vi "Teleop.vi"(10 "Match Info":T1={"Autonomous Elapsed Seconds"=0.0, "TeleOp Elapsed Seconds"=0.0, "Disabled Elapsed Seconds"=0.0, "Visited Autonomous"=FALSE, "Visited TeleOp"=FALSE, "Visited Disabled"=FALSE, "Autonomous Settings"={"Autonomous Style"=enum."Independent", "VI Refnum"=refnum}}, 11 "Call Context":T2=enum."Execute") -> ()   [LabVIEW 2013]
doc: "This VI is called for each TeleOp packet received from the DS where the robot is not disabled. It is often used to read from the joysticks and update I/O or to update setpoints for timed control loops. It should complete and return within 20 milliseconds or it may miss DS packets."
uses:
  <vilib>/Rock Robotics/WPI/DriverStation/WPI_DriverStationDerivedRobotMode.ctl
  <vilib>/Rock Robotics/WPI/DriverStation/WPI_DriverStationMatch Info.ctl
  Robot Global Data.vi
  <vilib>/Rock Robotics/WPI/Joystick/WPI_JoystickGetSetRefNum.vi
  <vilib>/Rock Robotics/WPI/RobotDrive/WPI_RobotDriveGetSetRefNum.vi
panel:
  in  "Joystick Mult Slow":dbl=0.5
  in  "Joystick Mult":dbl=1.0
  in  "Rest Speed r/s":dbl=15.0 min=0.0 max=0.7 step=0.05
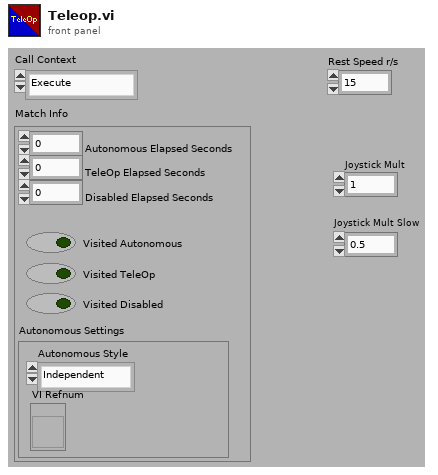
[diagram p1: front panel]
types:
  T1 = typedef "WPI_DriverStationMatch Info.ctl" = cluster{"Autonomous Elapsed Seconds":dbl, "TeleOp Elapsed Seconds":dbl, "Disabled Elapsed Seconds":dbl, "Visited Autonomous":bool, "Visited TeleOp":bool, "Visited Disabled":bool, "Autonomous Settings":cluster{"Autonomous Style":enum16{"Iterative", "Independent"}, "VI Refnum":refnum<vi>}}
  T2 = typedef "WPI_DriverStationDerivedRobotMode.ctl" = enum16{"Init", "Execute", "Stop"}
  T3 = typedef "WPI_JoystickDevRef.ctl" = cluster{"Device":T4}
  T4 = typedef "WPI_JoystickDeviceEnum.ctl" = enum16{"USB 1", "USB 2", "USB 3", "USB 4", "Kinect 1", "Kinect 2"}
  T5 = typedef "WPI_JoystickButtonState.ctl" = cluster{"Button 1":bool, "Button 2":bool, "Button 3":bool, "Button 4":bool, "Button 5":bool, "Button 6":bool, "Button 7":bool, "Button 8":bool, "Button 9":bool, "Button 10":bool, "Button 11":bool, "Button 12":bool}
  T6 = cluster{"axis 1 (x)":dbl, "axis 2 (y)":dbl, "axis 3 (throttle)":dbl, "axis 4":dbl, "axis 5":dbl, "axis 6":dbl}
  T7 = typedef "WPI_RobotDriveDevRef.ctl" = cluster{"DevStatus":errorcluster, "Motors[]":T8[], "Square Inputs":bool, "Max Output":dbl, "Isochronous":bool}
  T8 = typedef "WPI_MotorControlDeviceRef.ctl" = cluster{"DeviceStatus":errorcluster, "Type":enum16{"PWM", "CAN"}, "PWM":cluster{"Digital Module":T9, "PWM Channel":T10, "DeadBand":T11}, "CAN":cluster{"Device Number":u8, "Control Mode":T12, "Semaphore":T13, "Max Vout":dbl}, "Invert":bool, "TransformRef":T14, "InvTransformRef":T14}
  T9 = typedef "FPGA_TypedefDigitalModule.ctl" = enum16{"Digital Module 1", "Digital Module 2"}
  T10 = typedef "FPGA_DIOPWMChannel.ctl" = enum8{"PWM 1", "PWM 2", "PWM 3", "PWM 4", "PWM 5", "PWM 6", "PWM 7", "PWM 8", "PWM 9", "PWM 10", "Invalid"}
  T11 = typedef "WPI_PWMDeadband.ctl" = cluster{"Name":string, "maxPositivePwm":i32, "minPositivePwm":i32, "centerPwm":i32, "maxNegativePwm":i32, "minNegativePwm":i32, "angularRange":u16}
  T12 = typedef "WPI_CANJaguar_ControlMode.ctl" = enum8{"Percent VBus", "Current", "Speed", "Position", "Voltage"}
  T13 = typedef "Semaphore RefNum" = refnum<k1>
  T14 = typedef "WPI_PWMTransform_ConPane.ctl" = refnum<vi>
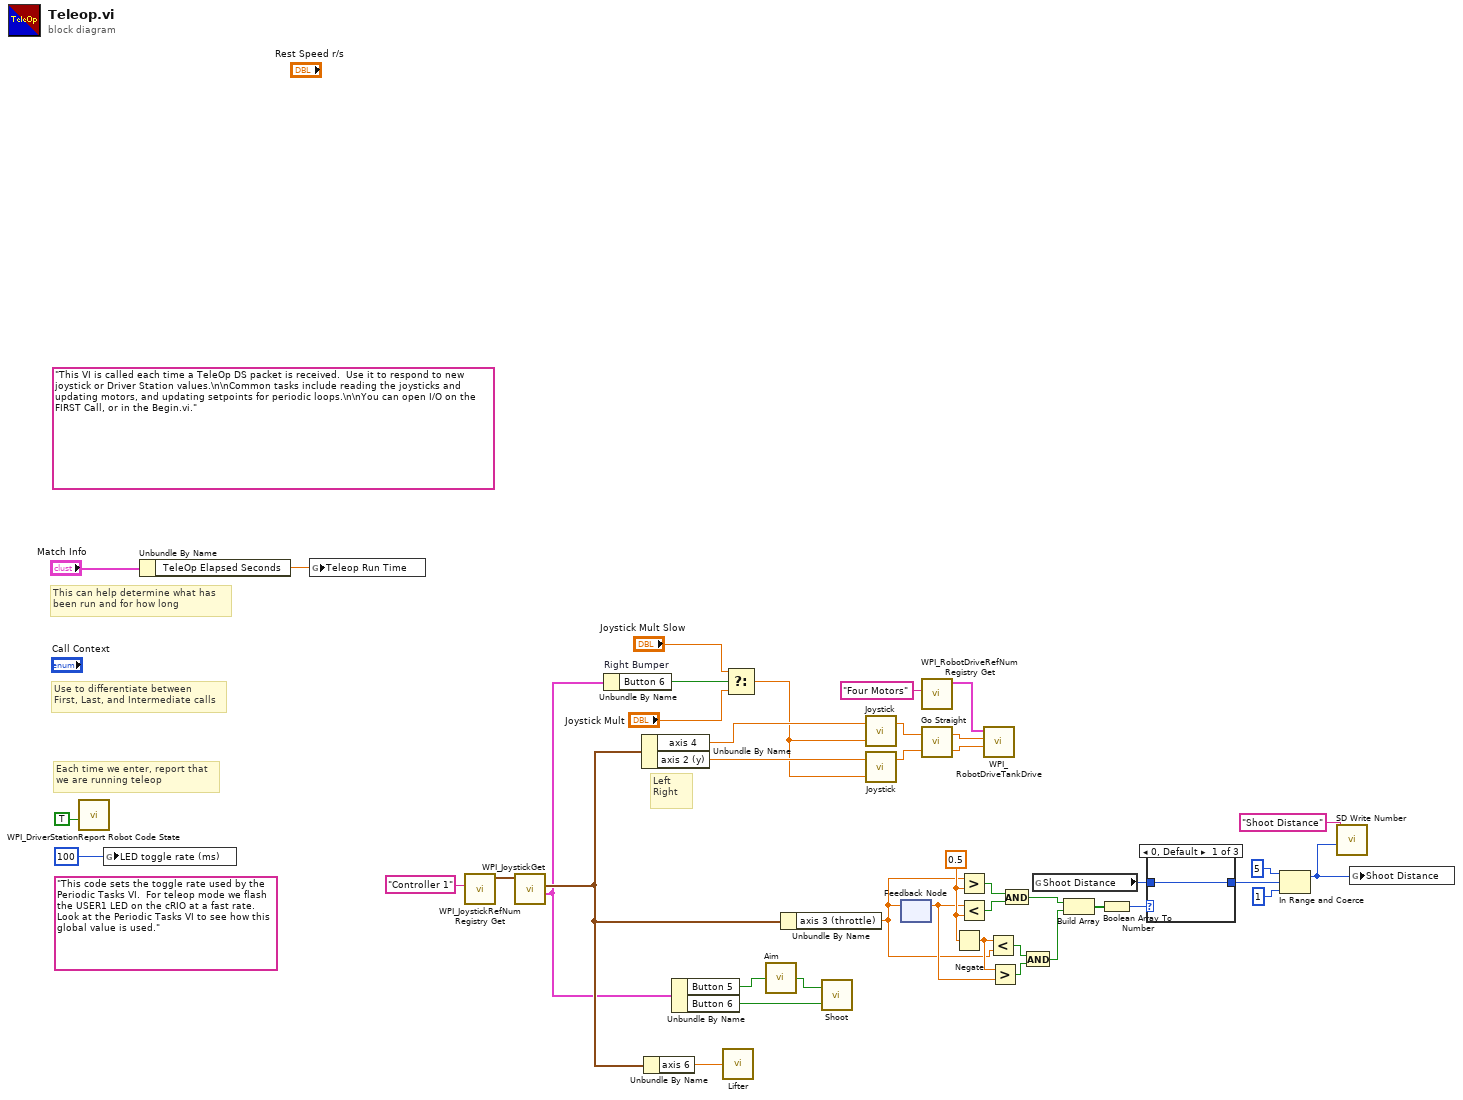
[diagram p0: block diagram]
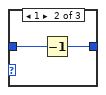
[diagram p2: hidden frame]
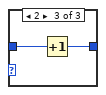
[diagram p3: hidden frame]
diagram:
  w31 = 0.5 ("y")
  (unwired) "This code sets the toggle rate used by the Periodic Tasks VI.  For teleop mode we flash the USER1 LED on the cRIO at a fast rate.  Look at the Periodic Tasks VI to see how this global value is used."
  (unwired) "This VI is called each time a TeleOp DS packet is received.  Use it to respond to new joystick or Driver Station values.\n\nCommon tasks include reading the joysticks and updating motors, and updating setpoints for periodic loops.\n\nYou can open I/O on the FIRST Call, or in the Begin.vi."
  # "Left\nRight"
  # "Each time we enter, report that\nwe are running teleop"
  # "Use to differentiate between\nFirst, Last, and Intermediate calls"
  # "This can help determine what has\nbeen run and for how long"
  n1 = call <vilib>:"WPI_DriverStationReport Robot Code State.vi"("TeleOp"=TRUE ("Autonomous")) -> ()  [unwired: 10 in, 1 out]
  n2 = global write "Robot Global Data.vi" "LED toggle rate (ms)"(u32 100 ("LED ms toggle rate")) -> ()
  n3 = Unbundle By Name("Match Info") -> ("TeleOp Elapsed Seconds"=w15:dbl)
  n4 = global write "Robot Global Data.vi" "Teleop Run Time"(w15) -> ()
  n5 = call <vilib>:"WPI_JoystickRefNum Registry Get.vi"("refnum name"="Controller 1") -> ("JoystickDevRef"=w40:T3)  [unwired: 1 in, 9 out]
  n6 = call <vilib>:"WPI_JoystickGet.vi"("JoystickDevRef"=w40) -> ("Buttons"=w2:T5, "Axes"=w3:T6)  [unwired: 1 in, 4 out]
  n7 = Unbundle By Name "Right Bumper"(w2) -> ("Button 6"=w37:bool)
  n8 = Unbundle By Name(w3) -> ("axis 4"=w12:dbl, "axis 2 (y)"=w11:dbl)
  n9 = Unbundle By Name(w3) -> ("axis 6"=w1:dbl)
  n10 = Unbundle By Name(w2) -> ("Button 5"=w9:bool, "Button 6"=w10:bool)
  n11 = call "Lifter.vi"("Joystick Speed"=w1) -> ()  [unwired: 1 out]
  n12 = Select(t="Joystick Mult Slow", s=w37, f="Joystick Mult") -> (s? t:f=w8:dbl)
  n13 = call "Aim.vi"("Aim"=w9) -> ("Ready"=w23:bool)
  n14 = Unbundle By Name(w3) -> ("axis 3 (throttle)"=w25:dbl)
  n15 = call "Shoot.vi"("Shoot"=w10, "Aiming"=w23) -> ()  [unwired: 1 out]
  n16 = call "Joystick.vi"("Multiplier"=w8, "Input"=w12) -> ("Output"=w7:dbl)  [unwired: 1 out]
  n17 = call "Joystick.vi"("Multiplier"=w8, "Input"=w11) -> ("Output"=w6:dbl)  [unwired: 1 out]
  n18 = feedback #1() -> (w29:dbl)  [unwired: 1 in]
  n19 = feedback-in #1(w25) -> ()
  n20 = call <vilib>:"WPI_RobotDriveRefNum Registry Get.vi"("refnum name"="Four Motors") -> ("RobotDriveDevRef"=w36:T7)  [unwired: 1 in, 9 out]
  n21 = call "Go Straight.vi"("Input Right"=w6, "Input Left"=w7) -> ("Output Right"=w4:dbl, "Output Left"=w5:dbl)
  n22 = Negate(x=w31) -> (-x=w30:dbl)
  n23 = Greater?(x=w25, y=w31) -> (0:w34:bool)
  n24 = Less?(x=w29, y=w31) -> (x < y?=w35:bool)
  n25 = call <vilib>:"WPI_RobotDriveTankDrive.vi"("Right axis value"=w4, "Left axis value"=w5, "RobotDriveDevRef"=w36) -> ()  [unwired: 6 in, 3 out]
  n26 = Less?(x=w30, y=w25) -> (x < y?=w32:bool)
  n27 = Greater?(x=w30, y=w29) -> (0:w33:bool)
  n28 = And(x=w34, y=w35) -> (x .and. y?=w28:bool)
  n29 = And(x=w32, y=w33) -> (x .and. y?=w27:bool)
  n30 = global read "Robot Global Data.vi" "Shoot Distance"() -> (w22:i32)
  n31 = Build Array(w28, w27) -> (w26:bool[])
  n32 = Boolean Array To Number(Boolean array=w26) -> (number=w24:u32)
  n33 = case shown="0, Default" w24 {
    tunnel: w22 -> [w43 w45 w47]
    tunnel: [w43 w44 w46] -> w21
    frame 0, Default {
    }
    frame 1 {
      n34 = Decrement(x=w45) -> (x-1=w44:i32)
    }
    frame 2 {
      n35 = Increment(x=w47) -> (x+1=w46:i32)
    }
  }
  n36 = In Range and Coerce(upper limit=5, x=w21, lower limit=1) -> (coerced(x)=w17:i32)  [unwired: 1 out]
  n37 = call <vilib>:"SD Write Number.vi"("Numeric"=w17, "Name"="Shoot Distance") -> ()  [unwired: 8 in, 2 out]
  n38 = global write "Robot Global Data.vi" "Shoot Distance"(w17) -> ()
